vi "输入对话框.vi"() -> ()   [LabVIEW 2013]
panel:
  out "年龄":dbl format="%#g"
  out "男":bool
  out "姓名":string
  in  "启用":bool
  in  "提示用户输入对话框":bool
  in  "退出":bool
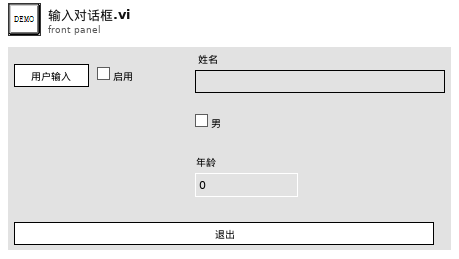
[diagram p1: front panel]
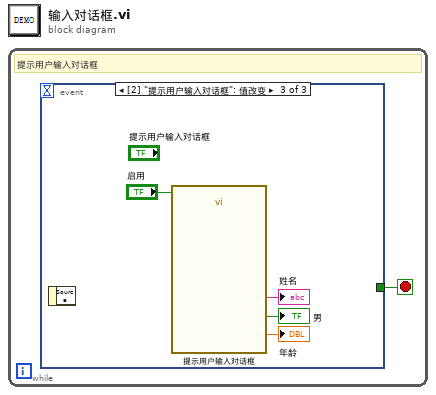
[diagram p0: block diagram]
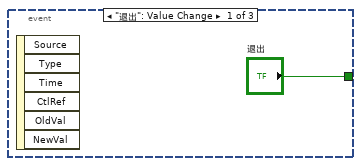
[diagram p2: hidden frame]
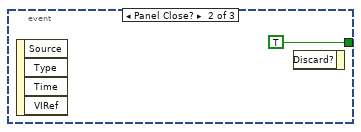
[diagram p3: hidden frame]
diagram:
  n1 = while {
    stop <- w1 stop-if-true
    # "提示用户输入对话框"
    n2 = event shown="[2] \"提示用户输入对话框\": 值改变" {
      selector: _ -> [_ _ _]
      dyn-events: _ -> [_ _ _]
      timeout: _ -> [_ _ _]
      tunnel: ["退出" TRUE ("退出") _] -> w1
      event "退出": Value Change {
        n3 = event-data() -> ()  [unwired: 1 in, 6 out]
      }
      event Panel Close? {
        n4 = event-data() -> ()  [unwired: 1 in, 4 out]
        n5 = event-data() -> ()  [unwired: 2 in, 1 out]
      }
      event "提示用户输入对话框": Value Change {
        n6 = event-data() -> ()  [unwired: 1 in, 1 out]
        n7 = call "提示用户输入对话框"("Enable"="启用") -> ("年龄"=→"年龄":dbl, "男"=→"男":bool, "姓名"=→"姓名":string)  [unwired: 14 in, 2 out]
      }
    }
  }
